vi "TestBed_timing.vi"() -> ()   [LabVIEW 2018]
uses:
  Types/method_enum.ctl
  HttpHeaders_response/HttpHeaders_Response.lvclass
  C:/Viviota/Projects/R&D/LabVIEW_HTTP_REST_NET/HTTPHeaders_NET/HttpHeaders_NET.lvclass
  HttpHeaders_content/HttpHeaders_Content.lvclass
  <vilib>/httpClient/Base64Encode.vi
  HttpHeaders_Request/HttpHeaders_Request.lvclass
  LabVIEWHTTPClient_NET/HttpClient_NET.lvclass
  HttpResponseMessage/HttpResponseMessage.lvclass
  HttpContent/HttpContent.lvclass
  HTTPHeaders_NET/HttpHeaders_NET.lvclass
  HttpClient_NET.lvlib
  HttpRequestMessage/HttpRequestMessage.lvclass
panel:
  in  "FilePath":path
  out "Content 2":u8[](array[numeric])
  out "Header Values 2":string[](array[string])
  out "Header Names 2":string[](array[string])
  out "error out":errorcluster
  in  "error in (no error)":errorcluster
  in  "URL":string="https://reqres.in/api/users?page=2"
  out "Content":string
  out "Header Names":string[](array[string])
  out "Header Values":string[](array[string])
  out "StatusCode":i32(ring)=100 items=["Continue"=100, "SwitchingProtocols"=101, "OK"=200, "Created"=201, "Accepted"=202, "NonAuthoritativeInformation"=203, "NoContent"=204, "ResetContent"=205, "PartialContent"=206, "MultipleChoices, Ambiguous"=300, "MovedPermanently, Moved"=301, "Found, Redirect"=302, "SeeOther, RedirectMethod"=303, "NotModified"=304, "UseProxy"=305, "Unused"=306, "TemporaryRedirect, RedirectKeepVerb"=307, "BadRequest"=400, "Unauthorized"=401, "PaymentRequired"=402, "Forbidden"=403, "NotFound"=404, "MethodNotAllowed"=405, "NotAcceptable"=406, "ProxyAuthenticationRequired"=407, "RequestTimeout"=408, "Conflict"=409, "Gone"=410, "LengthRequired"=411, "PreconditionFailed"=412, "RequestEntityTooLarge"=413, "RequestUriTooLong"=414, "UnsupportedMediaType"=415, "RequestedRangeNotSatisfiable"=416, "ExpectationFailed"=417, "UpgradeRequired"=426, "InternalServerError"=500, "NotImplemented"=501, "BadGateway"=502, "ServiceUnavailable"=503, "GatewayTimeout"=504, "HttpVersionNotSupported"=505]
  out "ReasonPhrase":string
  out "IsSuccessStatusCode":bool
  # "https://reqres.in/api/users?page=2"
  # "http://httpbin.org/basic-auth/user/password"
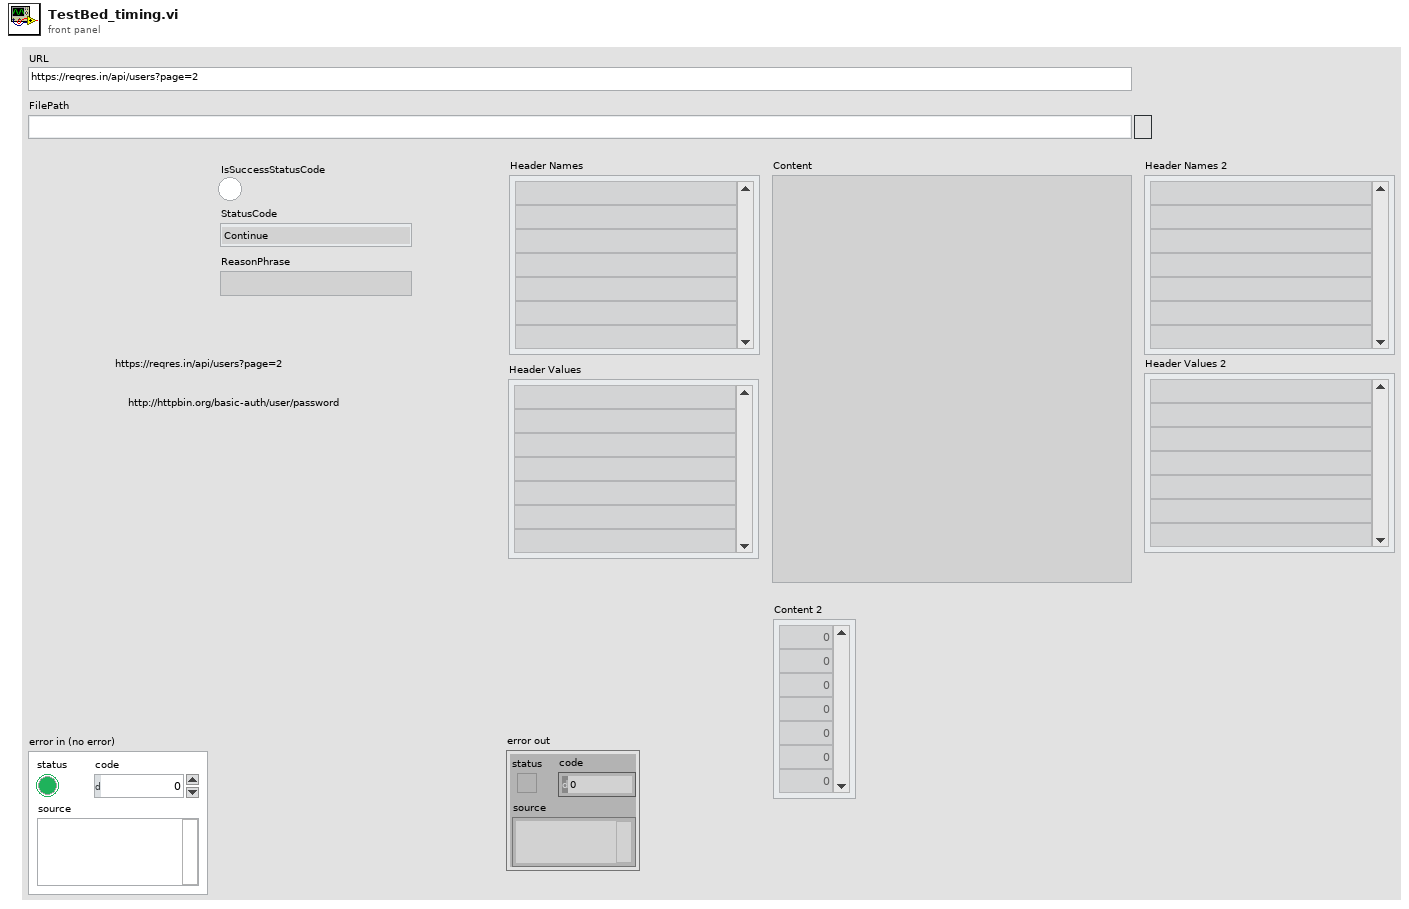
[diagram p1: front panel]
types:
  T1 = typedef "HttpClient_NET.lvlib/method_enum.ctl" = enum16{"GET", "PUT", "POST", "DELETE", "HEAD", "TRACE", "SEND"}
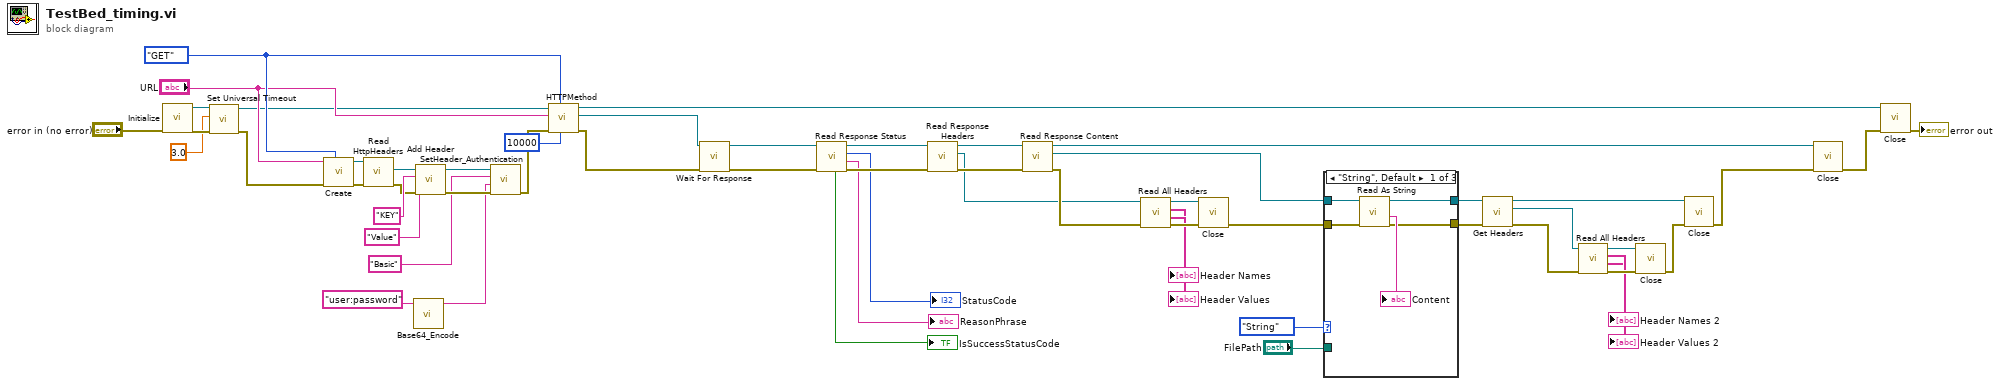
[diagram p0: block diagram]
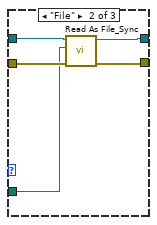
[diagram p2: hidden frame]
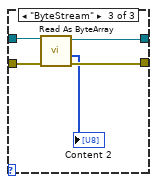
[diagram p3: hidden frame]
diagram:
  w25 = method_enum."GET" ("Method")
  n1 = call "Initialize.vi"("error in (no error)"="error in (no error)") -> ("error out"=w7:errorcluster, "HTTP Client Out"=w10:refnum<class "HttpClient_NET.lvclass">)  [unwired: 9 in]
  n2 = call "Set Universal Timeout.vi"("error in (no error)"=w7, "timeout_ms (10000)"=3.0 ("seconds [30]"), "LabVIEWHTTPClient_NET in"=w10) -> ("error out"=w8:errorcluster, "LabVIEWHTTPClient_NET out"=w9:refnum<class "HttpClient_NET.lvclass">)  [unwired: 7 in]
  n3 = call "Create.vi"("Method [GET]"=w25, "error in (no error)"=w8, "Address"="URL") -> ("error out"=w22:errorcluster, "HttpRequestMessage out"=w23:refnum<class "HttpRequestMessage.lvclass">)  [unwired: 7 in]
  n4 = call "Read HttpHeaders.vi"("error in (no error)"=w22, "HttpRequestMessage in"=w23) -> ("error out"=w19:errorcluster, "HttpHeaders"=w21:refnum<class "HttpHeaders_Request.lvclass">)  [unwired: 7 in, 1 out]
  n5 = call "Base64_Encode.vi"("buffer in"="user:password" ("scheme")) -> ("encoded string"=w12:string)  [unwired: 5 in, 1 out]
  n6 = call-dynamic "Add Header.vi"("error in (no error)"=w19, "Value"="Value", "Name"="KEY", "HTTPHeaders_NET in"=w21) -> ("error out"=w16:errorcluster, "HTTPHeaders_NET out"=w17:refnum<class "HttpHeaders_Request.lvclass">)  [unwired: 6 in]
  n7 = call "SetHeader_Authentication.vi"("error in (no error)"=w16, "parameter"=w12, "scheme"="Basic", "HttpHeaders_Request in"=w17) -> ("error out"=w15:errorcluster)  [unwired: 6 in, 1 out]
  n8 = call "HTTPMethod.vi"("Timeout_ms (10000)"=10000, "Method"=w25, "error in (no error)"=w15, "URL"="URL", "LabVIEWHTTPClient_NET in"=w9) -> ("error out"=w30:errorcluster, "HttpResponseMessage out"=w3:refnum<class "HttpResponseMessage.lvclass">, "LabVIEWHTTPClient_NET out"=w48:refnum<class "HttpClient_NET.lvclass">)  [unwired: 4 in]
  n9 = call "Wait For Response.vi"("error in (no error)"=w30, "HttpResponseMessage in"=w3) -> ("error out"=w4:errorcluster, "HttpResponseMessage out"=w2:refnum<class "HttpResponseMessage.lvclass">)  [unwired: 5 in, 3 out]
  n10 = call "Read Response Status.vi"("error in (no error)"=w4, "HttpResponseMessage in"=w2) -> ("error out"=w56:errorcluster, "ReasonPhrase"=→"ReasonPhrase":string, "StatusCode"=→"StatusCode":i32, "HttpResponseMessage out"=w57:refnum<class "HttpResponseMessage.lvclass">, "IsSuccessStatusCode"=→"IsSuccessStatusCode":bool)  [unwired: 4 in, 1 out]
  n11 = call "Read Response Headers.vi"("error in (no error)"=w56, "HttpResponseMessage in"=w57) -> ("error out"=w54:errorcluster, "HTTPHeaders_NET out"=w5:refnum<class "HttpHeaders_Response.lvclass">, "HttpResponseMessage out"=w55:refnum<class "HttpResponseMessage.lvclass">)  [unwired: 7 in]
  n12 = call "Read Response Content.vi"("error in (no error)"=w54, "HttpResponseMessage in"=w55) -> ("error out"=w29:errorcluster, "HttpContent out"=w53:refnum<class "HttpContent.lvclass">, "HttpResponseMessage out"=w49:refnum<class "HttpResponseMessage.lvclass">)  [unwired: 7 in]
  n13 = call-dynamic "Read All Headers.vi"("error in (no error)"=w29, "HTTPHeaders_NET in"=w5) -> ("error out"=w51:errorcluster, "Header Values"=→"Header Values":string[], "Header Names"=→"Header Names":string[], "HTTPHeaders_NET out"=w52:refnum<class "HttpHeaders_Response.lvclass">)  [unwired: 6 in]
  n14 = call "Close.vi"("error in (no error)"=w51, "HTTPHeaders_NET in"=w52) -> ("error out"=w50:errorcluster)  [unwired: 9 in]
  n15 = case shown="\"String\", Default" enum16{"String", "File", "ByteStream"}."String" {
    tunnel: w53 -> [w62 w65 w71]
    tunnel: [w60 w64 w70] -> w40
    tunnel: [w59 w66 w69] -> w39
    tunnel: w50 -> [w58 w67 w72]
    tunnel: "FilePath" -> [_ w63 _]
    frame "String", Default {
      n16 = call "Read As String.vi"("error in (no error)"=w58, "HttpContent in"=w62) -> ("error out"=w59:errorcluster, "Content"=→"Content":string, "HttpContent out"=w60:refnum<class "HttpContent.lvclass">)  [unwired: 7 in]
    }
    frame "File" {
      n17 = call "Read As File_Sync.vi"("error in (no error)"=w67, "FilePath"=w63, "HttpContent in"=w65) -> ("error out"=w66:errorcluster, "HttpContent out"=w64:refnum<class "HttpContent.lvclass">)  [unwired: 4 in, 3 out]
    }
    frame "ByteStream" {
      n18 = call "Read As ByteArray.vi"("error in (no error)"=w72, "HttpContent in"=w71) -> ("error out"=w69:errorcluster, "Content"=→"Content 2":u8[], "HttpContent out"=w70:refnum<class "HttpContent.lvclass">)  [unwired: 7 in]
    }
  }
  n19 = call "Get Headers.vi"("error in (no error)"=w39, "HttpContent in"=w40) -> ("error out"=w36:errorcluster, "HTTPHeaders"=w34:refnum<class "HttpHeaders_Content.lvclass">, "HttpContent out"=w33:refnum<class "HttpContent.lvclass">)  [unwired: 7 in]
  n20 = call-dynamic "Read All Headers.vi"("error in (no error)"=w36, "HTTPHeaders_NET in"=w34) -> ("error out"=w38:errorcluster, "Header Values"=→"Header Values 2":string[], "Header Names"=→"Header Names 2":string[], "HTTPHeaders_NET out"=w37:refnum<class "HttpHeaders_Content.lvclass">)  [unwired: 6 in]
  n21 = call "Close.vi"("error in (no error)"=w38, "HTTPHeaders_NET in"=w37) -> ("error out"=w35:errorcluster)  [unwired: 9 in]
  n22 = call "Close.vi"("error in (no error)"=w35, "HttpContent in"=w33) -> ("error out"=w28:errorcluster)  [unwired: 9 in]
  n23 = call "Close.vi"("error in (no error)"=w28, "HttpResponseMessage in"=w49) -> ("error out"=w47:errorcluster)  [unwired: 9 in]
  n24 = call "Close.vi"("Error In"=w47, "LabVIEWHTTPClient_NET in"=w48) -> ("Error Out"=→"error out":errorcluster)  [unwired: 9 in]
